vi "General Config.vi"(8 "error In":errorcluster, 10 "IOList":T2, 11 "reference":refnum<vi>) -> (0 "error out":errorcluster, 3 "Out reference":refnum<vi>)   [LabVIEW 2015]
uses:
  Control Button/Exit.ctl
  Control Button/Daq.ctl
  Control Button/Scanner config.ctl
  Control Button/Program Seq.ctl
  Control Button/cali.ctl
  Control Button/shift change.ctl
  Control Button/User mgt.ctl
  Control Button/model create.ctl
  Galobal variable_TI.vi
panel:
  out "Company Name  2":string
  in  "Image Setting":bool
  in  "Sensor Setting":bool
  out "User Name 3":string
  in  "Model Create":T1
  in  "User Mgt":T3
  out "User Name 2":string
  in  "Shift":T4
  in  "Calibration":T5
  in  "IO List Update":bool
  out "error out 2":errorcluster
  in  "error in (no error)":errorcluster
  in  "Program Seq":T6
  in  "Scanner config":T7
  in  "DAQ Config":T8
  out "User Name":string
  in  "Exit":T9
  out "String":string
  out "appended path":path
  in  "Ring":u16(ring)
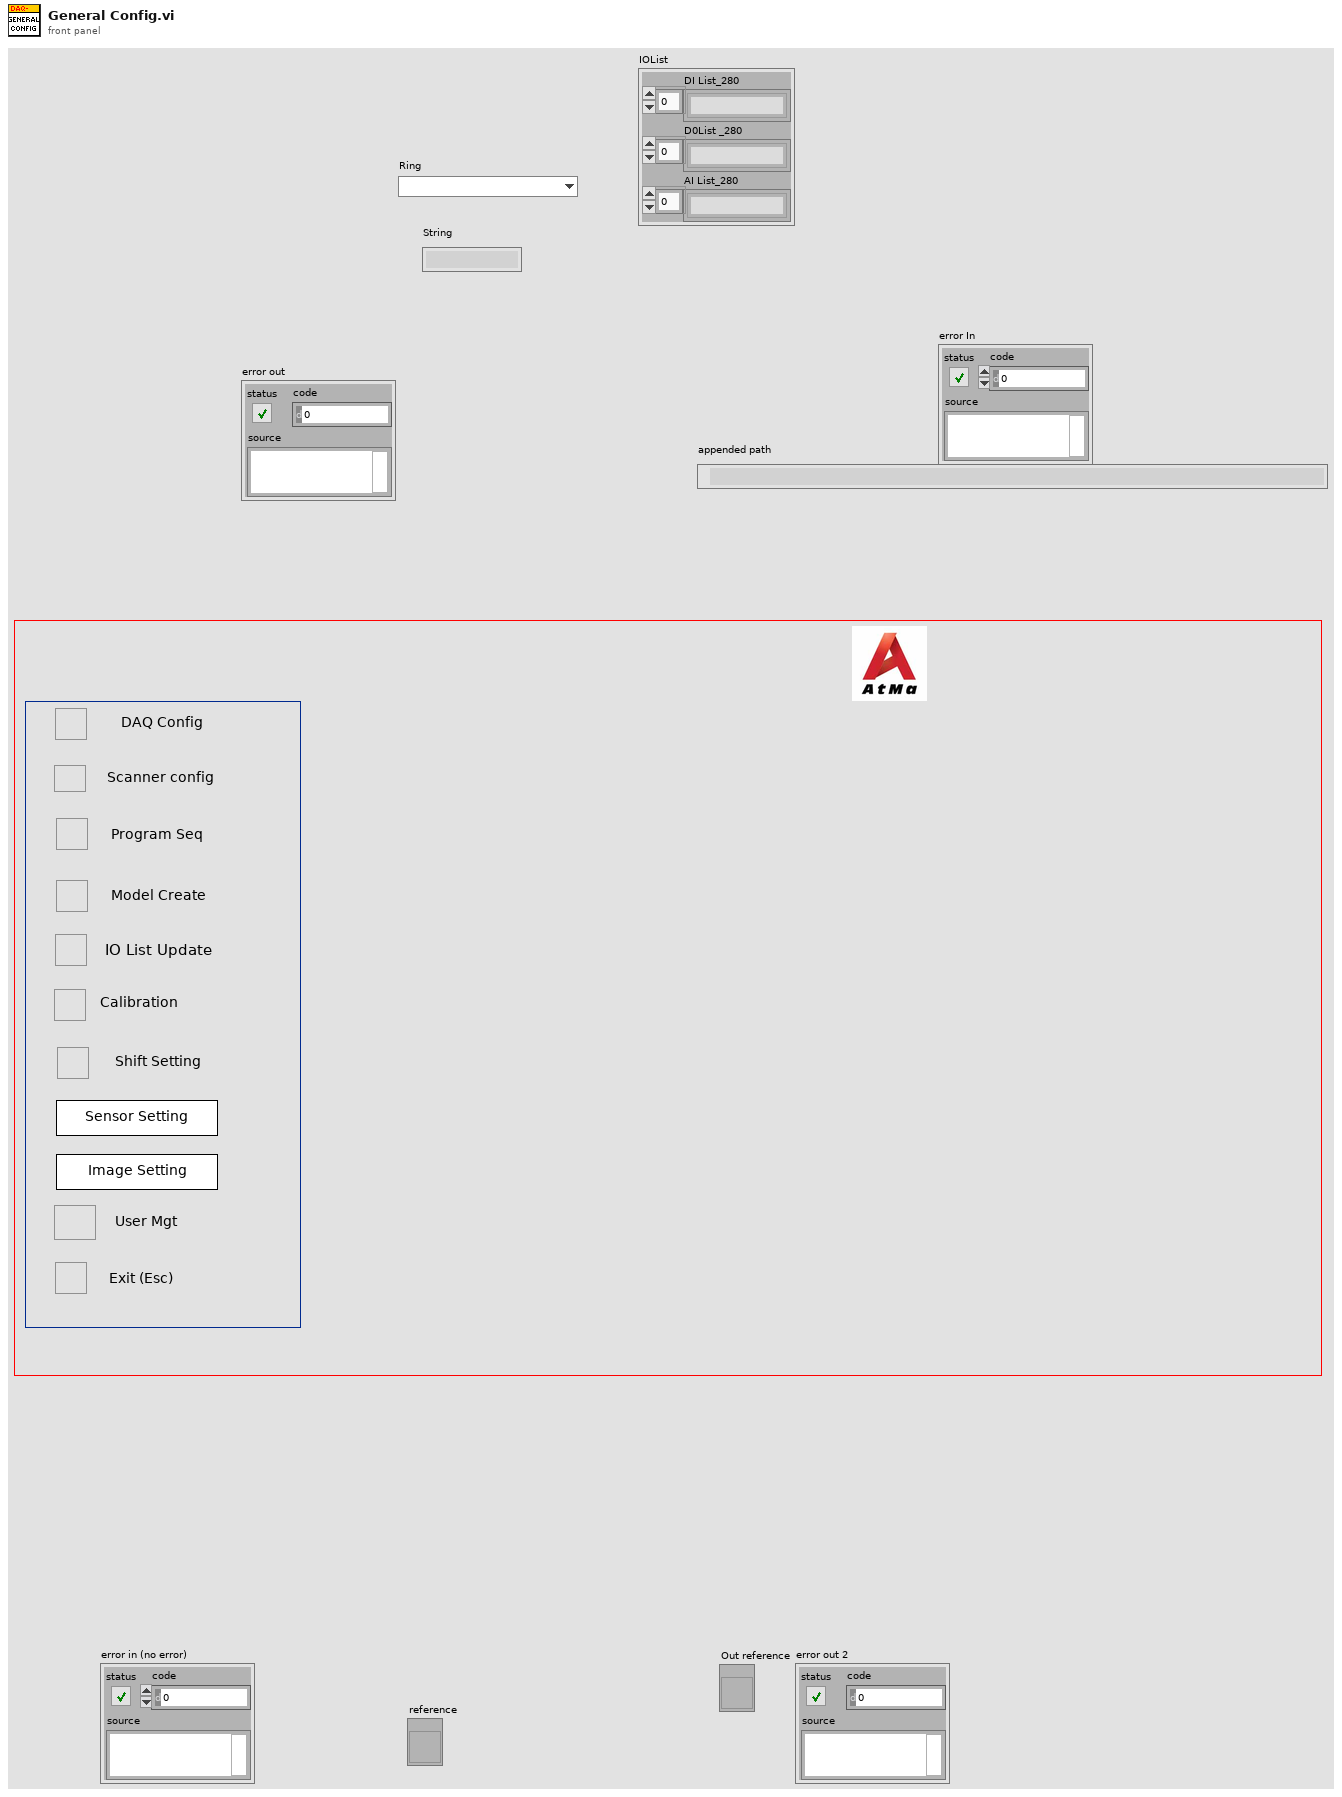
[diagram p1: front panel]
types:
  T1 = typedef "model create.ctl" = bool
  T2 = cluster{"DI List_280":string[], "D0List _280":string[], "AI List_280":string[]}
  T3 = typedef "User mgt.ctl" = bool
  T4 = typedef "shift change.ctl" = bool
  T5 = typedef "cali.ctl" = bool
  T6 = typedef "Program Seq.ctl" = bool
  T7 = typedef "Scanner config.ctl" = bool
  T8 = typedef "Daq.ctl" = bool
  T9 = typedef "Exit.ctl" = bool
  T10 = enum32{"Invalid", "Standard", "Closed", "Hidden", "Minimized", "Maximized"}
  T11 = cluster{"XInput":dbl[], "Y New Value":dbl[], "Avg point":i16}[]
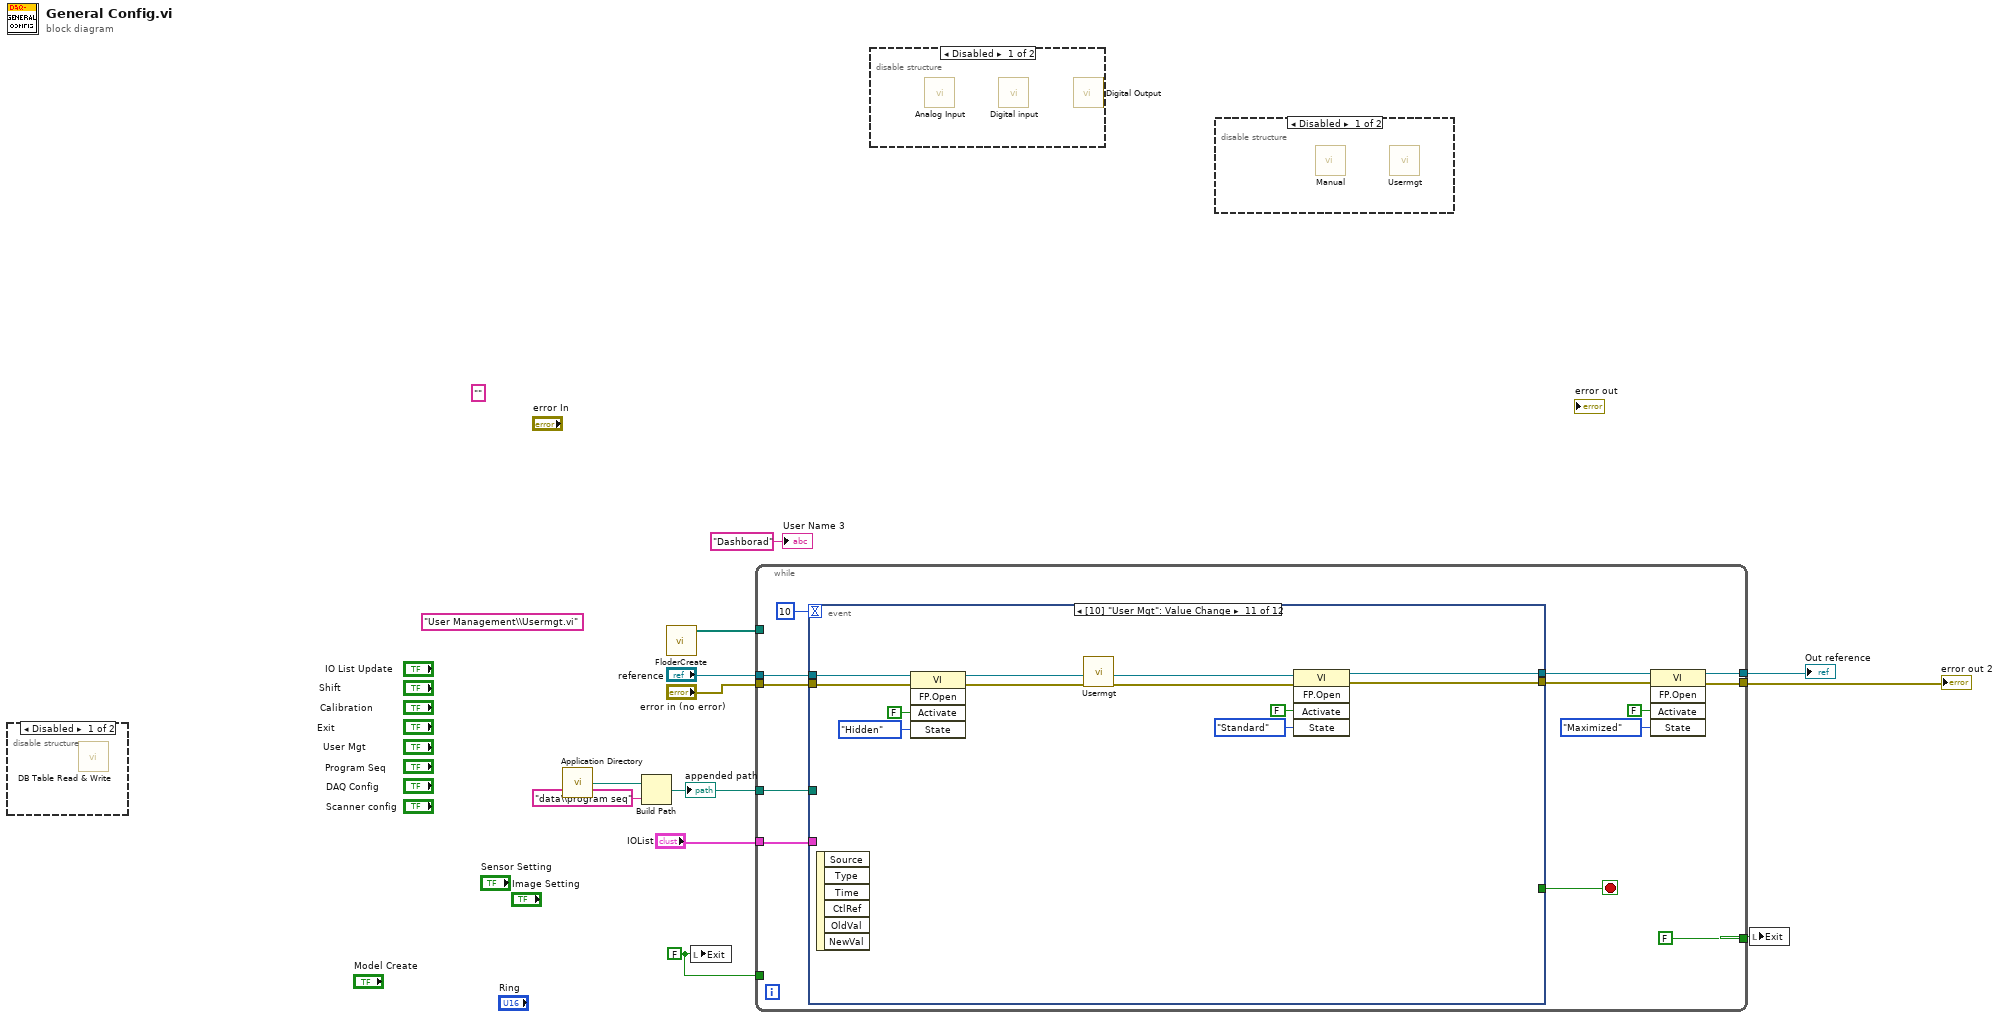
[diagram p0: block diagram]
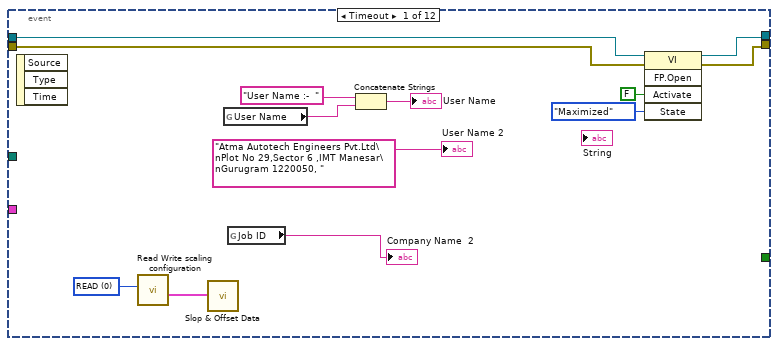
[diagram p5: hidden frame]
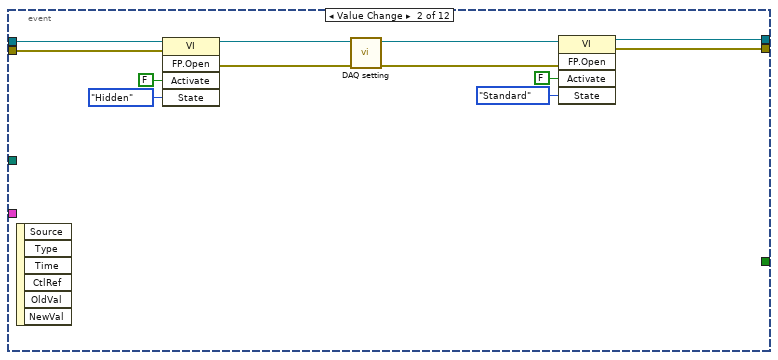
[diagram p6: hidden frame]
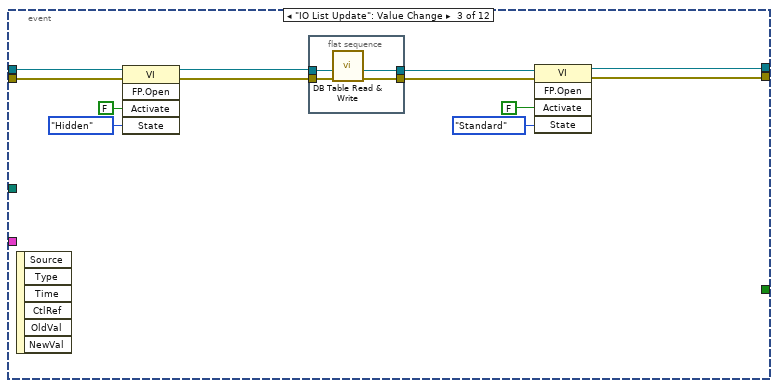
[diagram p7: hidden frame]
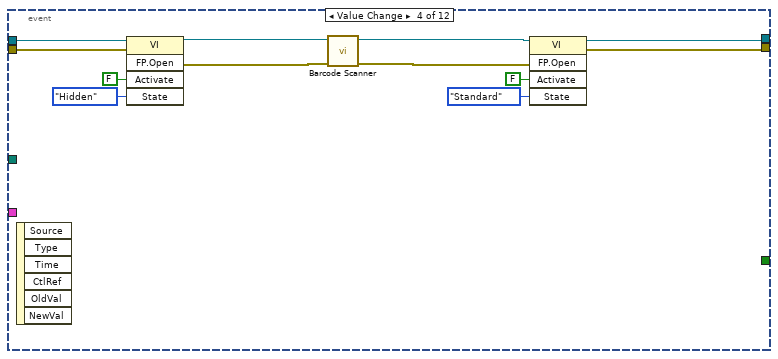
[diagram p8: hidden frame]
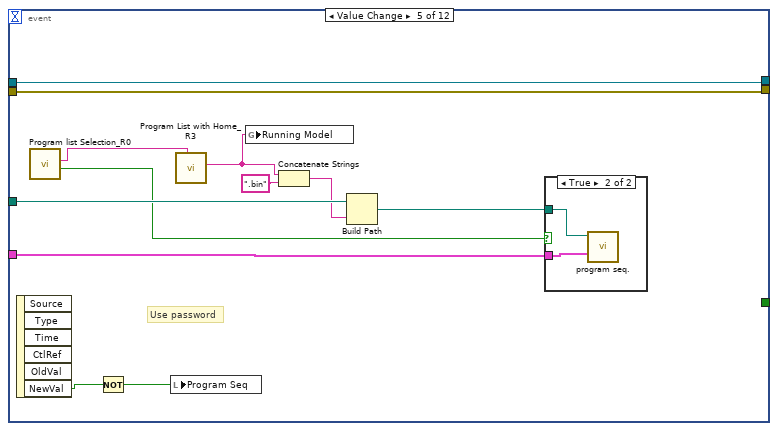
[diagram p9: hidden frame]
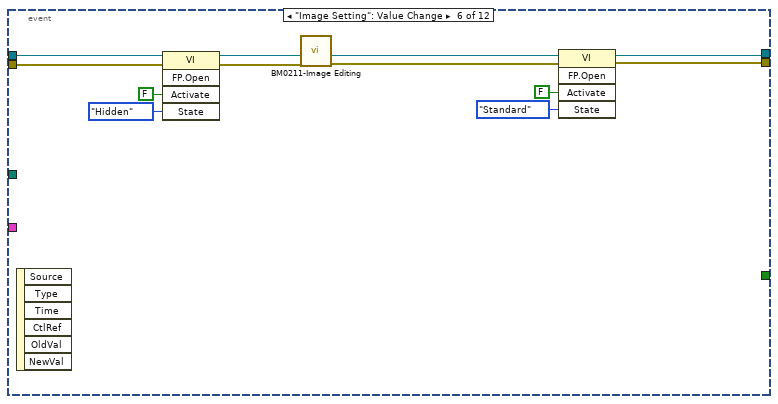
[diagram p11: hidden frame]
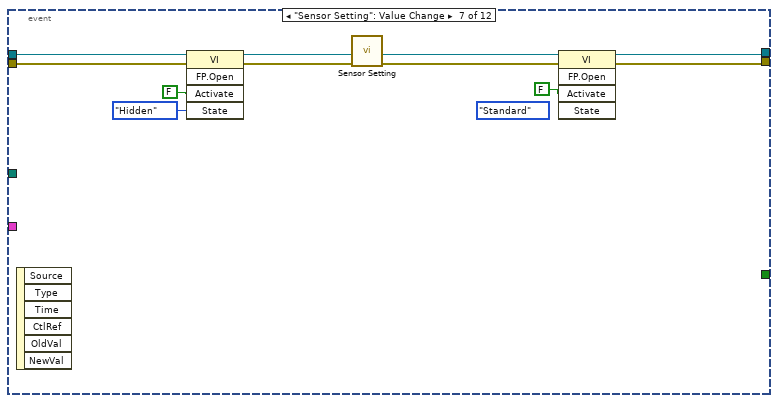
[diagram p12: hidden frame]
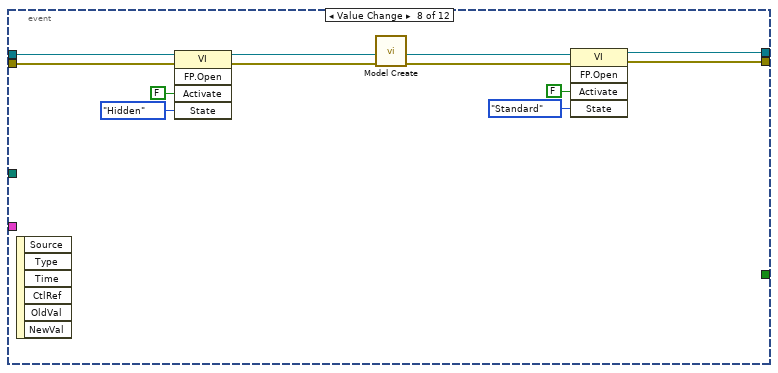
[diagram p13: hidden frame]
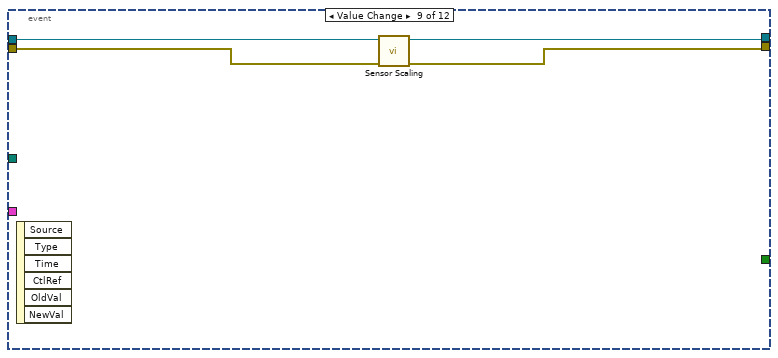
[diagram p14: hidden frame]
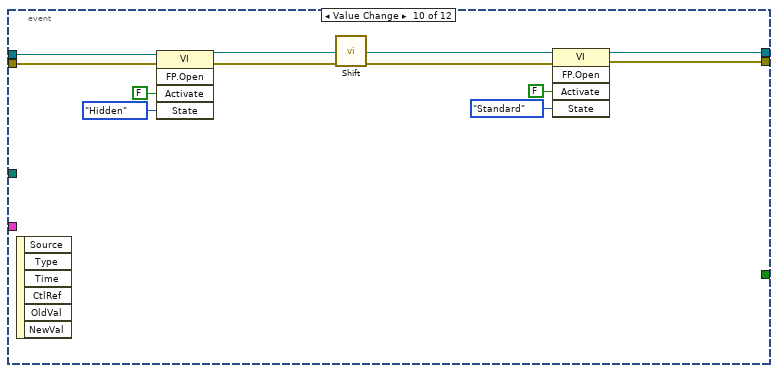
[diagram p15: hidden frame]
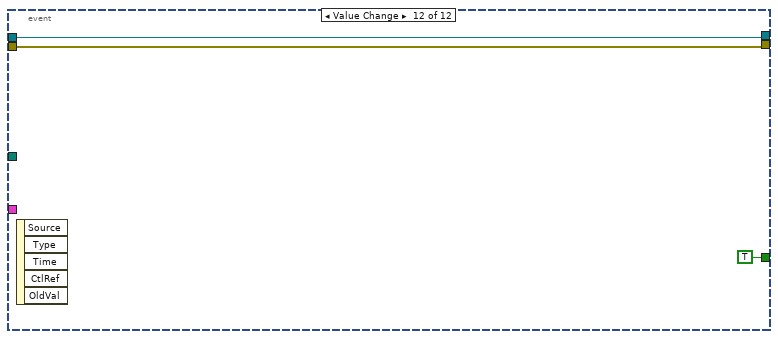
[diagram p16: hidden frame]
diagram:
  w9 = T9 FALSE ("Exit")
  (unwired) "User Management\\Usermgt.vi" ("name or relative path")
  (unwired) ""
  n1 = disable-structure shown="Disabled" {
    frame Disabled {
      n2 = call "DB Table Read & Write.vi"() -> ()  [unwired: 10 in, 2 out]
    }
    frame Enabled {
    }
  }
  n3 = call <vilib>:"Application Directory.vi"() -> ("Application Directory"=w5:path)
  n4 = Build Path(base path=w5, name or relative path="data\\program seq") -> (appended path=w2:path)
  "appended path" <- w2
  n5 = call "FloderCreate.vi"() -> ("File Path"=w6:path[])  [unwired: 11 in]
  n6 = local write "Exit"(w9) -> ()
  n7 = while {
    tunnel: w2 -> [w13]
    tunnel: "reference" -> [w23]
    tunnel: "error in (no error)" -> [w22]
    tunnel: [w17] -> w11
    tunnel: [w16] -> w10
    tunnel: w9 -> [_]
    tunnel: [T9 FALSE ("Exit")] -> w8
    tunnel: w6 -> [_]
    tunnel: "IOList" -> [w14]
    stop <- w24 stop-if-true
    n8 = event shown="[10] \"User Mgt\": Value Change" {
      selector: _ -> [_ _ _ _ _ _ _ _ _ _ _ _]
      dyn-events: _ -> [_ _ _ _ _ _ _ _ _ _ _ _]
      timeout: 10 -> [_ _ _ _ _ _ _ _ _ _ _ _]
      tunnel: [_ _ _ _ _ _ _ _ _ _ _ TRUE ("Exit")] -> w24
      tunnel: w23 -> [w29 w42 w54 w76 w90 w101 w108 w118 w125 w133 w142 w150]
      tunnel: w22 -> [w27 w41 w53 w75 w89 w94 w107 w117 w124 w131 w140 w149]
      tunnel: [w28 w40 w61 w72 w90 w101 w103 w113 w125 w132 w141 w150] -> w19
      tunnel: [w26 w39 w60 w71 w89 w93 w102 w112 w123 w130 w139 w149] -> w18
      tunnel: w14 -> [_ _ _ _ w88 _ _ _ _ _ _ _]
      tunnel: w13 -> [_ _ _ _ w87 _ _ _ _ _ _ _]
      event Timeout {
        w35 = u16 0 items=["READ", "WRITE"] ("Read/Write")
        n9 = event-data() -> ()  [unwired: 1 in, 3 out]
        n10 = call "Read Write scaling configuration.vi"("Read/Write"=w35) -> ("Output"=w34:T11)  [unwired: 4 in, 2 out]
        n11 = call "Slop & Offset Data.vi"("Input"=w34) -> ()  [unwired: 10 in, 1 out]
        n12 = global read "Galobal variable_TI.vi" "User Name"() -> (w38:string)
        n13 = global read "Galobal variable_TI.vi" "Job ID"() -> (→"Company Name  2":string)
        n14 = Concatenate Strings("User Name :-  " ("string"), w38) -> (→"User Name":string)
        n15 = invoke class="VI" method="FP.Open"(reference=w29, error in=w27, "Activate"=FALSE ("Activate?"), "State"=T10."Maximized") -> (reference out=w28:refnum<vi>, error out=w26:errorcluster)  [unwired: 1 in, 3 out]
        "User Name 2" <- "Atma Autotech Engineers Pvt.Ltd\nPlot No 29,Sector 6 ,IMT Manesar\nGurugram 1220050, " ("string")
      }
      event Value Change {
        n16 = event-data() -> ()  [unwired: 1 in, 6 out]
        n17 = invoke class="VI" method="FP.Open"(reference=w42, error in=w41, "Activate"=FALSE ("Activate?"), "State"=T10."Hidden") -> (reference out=w48:refnum<vi>, error out=w47:errorcluster)  [unwired: 1 in, 3 out]
        n18 = call "DAQ setting.vi"("error in (no error)"=w47, "vi reference"=w48) -> ("error Out"=w43:errorcluster, "Out reference"=w44:refnum<vi>)  [unwired: 8 in]
        n19 = invoke class="VI" method="FP.Open"(reference=w44, error in=w43, "Activate"=FALSE ("Activate?"), "State"=T10."Standard") -> (reference out=w40:refnum<vi>, error out=w39:errorcluster)  [unwired: 1 in, 3 out]
      }
      event "IO List Update": Value Change {
        n20 = event-data() -> ()  [unwired: 1 in, 6 out]
        n21 = invoke class="VI" method="FP.Open"(reference=w54, error in=w53, "Activate"=FALSE ("Activate?"), "State"=T10."Hidden") -> (reference out=w52:refnum<vi>, error out=w51:errorcluster)  [unwired: 1 in, 3 out]
        n22 = flat-sequence {
          tunnel: [w63] -> w58
          tunnel: [w64] -> w57
          tunnel: w52 -> [w65]
          tunnel: w51 -> [w66]
          frame #0 {
            n23 = call "DB Table Read & Write.vi"("error in"=w66, "reference"=w65) -> ("error out"=w63:errorcluster, "referenceOut"=w64:refnum<vi>)  [unwired: 8 in]
          }
        }
        n24 = invoke class="VI" method="FP.Open"(reference=w57, error in=w58, "Activate"=FALSE ("Activate?"), "State"=T10."Standard") -> (reference out=w61:refnum<vi>, error out=w60:errorcluster)  [unwired: 1 in, 3 out]
      }
      event Value Change {
        n25 = event-data() -> ()  [unwired: 1 in, 6 out]
        n26 = invoke class="VI" method="FP.Open"(reference=w76, error in=w75, "Activate"=FALSE ("Activate?"), "State"=T10."Hidden") -> (reference out=w68:refnum<vi>, error out=w70:errorcluster)  [unwired: 1 in, 3 out]
        n27 = call "Barcode Scanner.vi"("error in (no error)"=w70, "reference"=w68) -> ("error in (no error) 2"=w69:errorcluster, "reference 2"=w67:refnum<vi>)  [unwired: 8 in]
        n28 = invoke class="VI" method="FP.Open"(reference=w67, error in=w69, "Activate"=FALSE ("Activate?"), "State"=T10."Standard") -> (reference out=w72:refnum<vi>, error out=w71:errorcluster)  [unwired: 1 in, 3 out]
      }
      event Value Change {
        # "Use password"
        n29 = event-data() -> ("NewVal"=w82:T6)  [unwired: 1 in, 5 out]
        n30 = call "Program list Selection_R0.vi"() -> ("Exit"=w83:bool, "String"=w80:string)  [unwired: 8 in, 2 out]
        n31 = Not(x=w82) -> (.not. x?=w81:T6)
        n32 = local write "Program Seq"(w81) -> ()
        n33 = call "Program List with Home_R3.vi"("Model"=w80) -> ("String"=w79:string)  [unwired: 7 in, 3 out]
        n34 = global write "Galobal variable_TI.vi" "Running Model"(w79) -> ()
        n35 = Concatenate Strings(w79, ".bin" ("string")) -> (w86:string)
        n36 = Build Path(base path=w87, name or relative path=w86) -> (appended path=w84:path)
        n37 = case shown="True" w83 {
          tunnel: w88 -> [_ w91]
          tunnel: w84 -> [_ w92]
          frame False {
          }
          frame True {
            n38 = call "program seq..vi"("IOList"=w91, "Filepath"=w92) -> ()  [unwired: 9 in, 1 out]
          }
        }
      }
      event "Image Setting": Value Change {
        n39 = event-data() -> ()  [unwired: 1 in, 6 out]
        n40 = invoke class="VI" method="FP.Open"(error in=w94, "Activate"=FALSE ("Activate?"), "State"=T10."Hidden") -> (error out=w96:errorcluster)  [unwired: 2 in, 4 out]
        n41 = call "BM0211-Image Editing.vi"("error IN"=w96) -> ("error out"=w95:errorcluster)  [unwired: 10 in]
        n42 = invoke class="VI" method="FP.Open"(error in=w95, "Activate"=FALSE ("Activate?"), "State"=T10."Standard") -> (error out=w93:errorcluster)  [unwired: 2 in, 4 out]
      }
      event "Sensor Setting": Value Change {
        (unwired) T10."Standard" ("State")
        n43 = event-data() -> ()  [unwired: 1 in, 6 out]
        n44 = invoke class="VI" method="FP.Open"(reference=w108, error in=w107, "Activate"=FALSE ("Activate?"), "State"=T10."Hidden") -> (reference out=w104:refnum<vi>, error out=w106:errorcluster)  [unwired: 1 in, 3 out]
        n45 = call "Sensor Setting.vi"("error in"=w106) -> ("error  out"=w105:errorcluster)  [unwired: 10 in]
        n46 = invoke class="VI" method="FP.Open"(reference=w104, error in=w105, "Activate"=FALSE ("Activate?")) -> (reference out=w103:refnum<vi>, error out=w102:errorcluster)  [unwired: 2 in, 3 out]
      }
      event Value Change {
        n47 = event-data() -> ()  [unwired: 1 in, 6 out]
        n48 = invoke class="VI" method="FP.Open"(reference=w118, error in=w117, "Activate"=FALSE ("Activate?"), "State"=T10."Hidden") -> (reference out=w114:refnum<vi>, error out=w116:errorcluster)  [unwired: 1 in, 3 out]
        n49 = call "Model Create.vi"("error in (no error)"=w116) -> ("error out"=w115:errorcluster)  [unwired: 10 in]
        n50 = invoke class="VI" method="FP.Open"(reference=w114, error in=w115, "Activate"=FALSE ("Activate?"), "State"=T10."Standard") -> (reference out=w113:refnum<vi>, error out=w112:errorcluster)  [unwired: 1 in, 3 out]
      }
      event Value Change {
        n51 = event-data() -> ()  [unwired: 1 in, 6 out]
        n52 = call "Sensor Scaling.vi"("error in"=w124) -> ("error out"=w123:errorcluster)  [unwired: 9 in, 1 out]
      }
      event Value Change {
        n53 = event-data() -> ()  [unwired: 1 in, 6 out]
        n54 = invoke class="VI" method="FP.Open"(reference=w133, error in=w131, "Activate"=FALSE ("Activate?"), "State"=T10."Hidden") -> (reference out=w134:refnum<vi>, error out=w136:errorcluster)  [unwired: 1 in, 3 out]
        n55 = call "Shift.vi"("error in"=w136) -> ("error out"=w135:errorcluster)  [unwired: 10 in]
        n56 = invoke class="VI" method="FP.Open"(reference=w134, error in=w135, "Activate"=FALSE ("Activate?"), "State"=T10."Standard") -> (reference out=w132:refnum<vi>, error out=w130:errorcluster)  [unwired: 1 in, 3 out]
      }
      event Value Change {
        n57 = event-data() -> ()  [unwired: 1 in, 6 out]
        n58 = invoke class="VI" method="FP.Open"(reference=w142, error in=w140, "Activate"=FALSE ("Activate?"), "State"=T10."Hidden") -> (reference out=w143:refnum<vi>, error out=w138:errorcluster)  [unwired: 1 in, 3 out]
        n59 = call "Usermgt.vi"("error In"=w138) -> ("error out"=w137:errorcluster)  [unwired: 10 in]
        n60 = invoke class="VI" method="FP.Open"(reference=w143, error in=w137, "Activate"=FALSE ("Activate?"), "State"=T10."Standard") -> (reference out=w141:refnum<vi>, error out=w139:errorcluster)  [unwired: 1 in, 3 out]
      }
      event Value Change {
        n61 = event-data() -> ()  [unwired: 1 in, 5 out]
      }
    }
    n62 = invoke class="VI" method="FP.Open"(reference=w19, error in=w18, "Activate"=FALSE ("Activate?"), "State"=T10."Maximized") -> (reference out=w17:refnum<vi>, error out=w16:errorcluster)  [unwired: 1 in, 3 out]
  }
  "Out reference" <- w11
  "error out 2" <- w10
  n63 = disable-structure shown="Disabled" {
    frame Disabled {
      n64 = call "Analog Input.vi"() -> ()  [unwired: 10 in, 2 out]
      n65 = call "Digital input.vi"() -> ()  [unwired: 10 in, 2 out]
      n66 = call "Digital Output.vi"() -> ()  [unwired: 10 in, 2 out]
    }
    frame Enabled {
    }
  }
  n67 = disable-structure shown="Disabled" {
    frame Disabled {
      n68 = call "Manual.vi"() -> ()  [unwired: 10 in, 2 out]
      n69 = call "Usermgt.vi"() -> ()  [unwired: 11 in, 1 out]
    }
    frame Enabled {
    }
  }
  n70 = local write "Exit"(w8) -> ()
  "User Name 3" <- "Dashborad" ("User Name 3")
